vi "GetPlots.vi"(8 "error in":errorcluster, 11 "WaveformChart in":refnum<class "WaveformChart.lvclass">) -> (0 "error out":errorcluster, 3 "WaveformChart out":refnum<class "WaveformChart.lvclass">)   [LabVIEW 2014, in "Raspberry Pi Compatible Compiler for LabVIEW.lvlib" / "WaveformChart.lvclass"]
uses:
  WaveformChart.lvclass
  WaveformChart.lvclass/WaveformChart.ctl
  Plot/Plot.lvclass
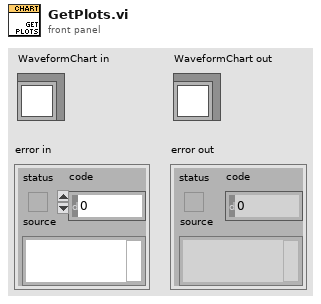
[diagram p1: front panel]
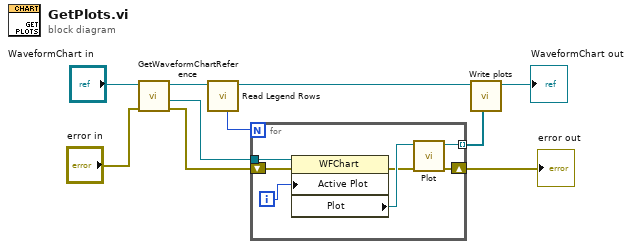
[diagram p0: block diagram]
diagram:
  n1 = call "GetWaveformChartReference.vi"("error in"="error in", "WFChart in"="WaveformChart in") -> ("error out"=w9:errorcluster, "graph scale reference"=w8:refnum<vi>, "WFChart out"=w6:refnum<class "WaveformChart.lvclass">)  [unwired: 7 in]
  n2 = call "Read Legend Rows.vi"("WaveformChart in"=w6) -> ("WaveformChart out"=w4:refnum<class "WaveformChart.lvclass">, "Legend Rows"=w10:u32)  [unwired: 7 in]
  n3 = for {
    N: w10 -> [_]
    shift-right: [w12] -> w2
    shift-left: w9 -> [w17]
    tunnel: w8 -> [w16]
    tunnel: [w11] -> w7 mode=indexing
    i -> [w15]
    n4 = property class="WFChart"(reference=w16, error in=w17, "Active Plot"=w15) -> (error out=w13:errorcluster, "Plot"=w14:refnum<vi>)  [unwired: 1 out]
    n5 = call "Plot.vi"("error in"=w13, "Plot Refnum"=w14) -> ("error out"=w12:errorcluster, "Plot out"=w11:refnum<class "Plot.lvclass">)  [unwired: 8 in]
  }
  "error out" <- w2
  n6 = call "Write plots.vi"("plots"=w7, "WaveformChart in"=w4) -> ("WaveformChart out"=→"WaveformChart out":refnum<class "WaveformChart.lvclass">)  [unwired: 7 in]
